vi "7thOrderExpandedWLC.FitFunc.vi"(3 "output control":T1, 4 "data":variant, 5 "X":dbl[](array[numeric]), 6 "Coefficients":dbl[](array[numeric])) -> (0 "error out":errorcluster, 1 "f'(X,a)":dbl[][](array[numeric]), 2 "f(X,a)":dbl[](array[numeric]))   [LabVIEW 2020, in "XYcenter.lvlib"]
uses:
  XYcenter.lvlib
  <vilib>/gmath/NumericalOptimization/LM_output select.ctl
  <vilib>/gmath/NI_Gmath.lvlib
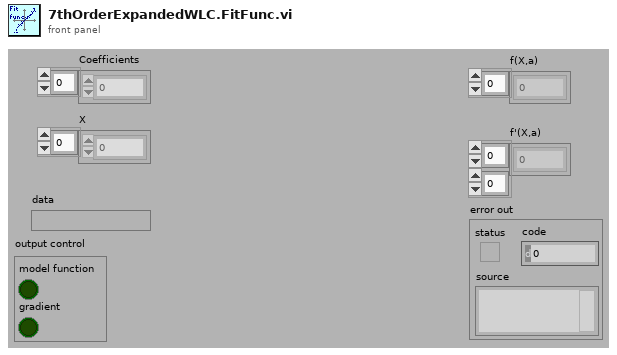
[diagram p1: front panel]
types:
  T1 = typedef "NI_Gmath.lvlib/LM_output select.ctl" = cluster{"model function":bool, "gradient":bool}
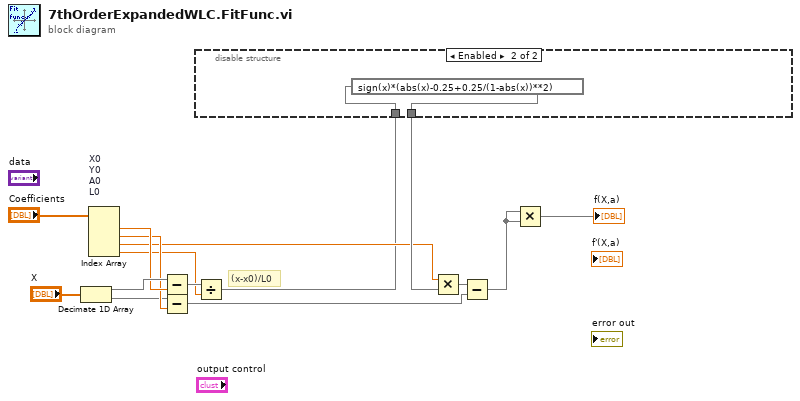
[diagram p0: block diagram]
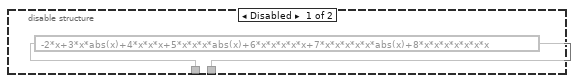
[diagram p2: hidden frame]
diagram:
  # "(x-x0)/L0"
  n1 = Decimate 1D Array("X") -> (w13:dbl[], w10:dbl[])
  n2 = Index Array "X0\nY0\nA0\nL0"(array="Coefficients") -> (element #1=w12:dbl, element #2=w11:dbl, element #3=w8:dbl, element #4=w6:dbl)  [unwired: 4 in]
  n3 = Subtract(x=w13, y=w12) -> (x-y=w7:dbl[])
  n4 = Subtract(x=w10, y=w11) -> (x-y=w4:dbl[])
  n5 = Divide(x=w7, y=w6) -> (x/y=w1:dbl[])
  n6 = disable-structure shown="Enabled" {
    disable-tunnel: [w17 w18] -> w9
    disable-tunnel: w1 -> [w16 w19]
    frame Disabled {
      n7 = expression code="-2*x+3*x*abs(x)+4*x*x*x+5*x*x*x*abs(x)+6*x*x*x*x*x+7*x*x*x*x*x*abs(x)+8*x*x*x*x*x*x*x"(w16) -> (w17:dbl[])
    }
    frame Enabled {
      n8 = expression code="sign(x)*(abs(x)-0.25+0.25/(1-abs(x))**2)"(w19) -> (w18:dbl[])
    }
  }
  n9 = Multiply(x=w8, y=w9) -> (x*y=w5:dbl[])
  n10 = Subtract(x=w5, y=w4) -> (x-y=w2:dbl[])
  n11 = Multiply(x=w2, y=w2) -> (x*y=→"f(X,a)":dbl[])
